vi "GeneratorBiasCurrents.vi"(10 "CurrentWaveForm":T1={"StartCurrent (mA)"=1.0, "MaximumCurrent (mA)"=3.0, "NumberOfCurrentPoints"=3, "NumberOfPointsInPulse"=20, "NumOfPointsAtPulseMAX"=4, "Exponent"=1, "CurrentStep (mA)"=1.0, "NumOfPointsAtPulseMIN"=8, "Next current step"=0.0} {"StartCurrent (mA)" min=0.001}) -> (0 "PulsedCurrentWaveForm":dbl[](array[numeric])=[0.0, 0.0, 0.0, 0.0, 0.0, 0.0, 0.0, 0.0, 0.0, 0.006819348298638839, 0.02709137914968268, 0.06026312439675552, 0.10542974530180321, 0.16135921418712945, 0.22652592093878654, 0.29915228767351526, 0.3772572564296004, 0.4587103272638338, 0.5412896727361661, 0.6227427435703996, 0.7008477123264847, 0.7734740790612133, 0.8386407858128705, 0.8945702546981968, 0.9397368756032445, 0.9729086208503173, 0.9931806517013612, 1.0, 1.0, 1.0, 1.0, 1.0, 1.0, 0.9931806517013612, 0.9729086208503173, 0.9397368756032445, 0.8945702546981968, 0.8386407858128706, 0.7734740790612135, 0.7008477123264847, 0.6227427435703996, 0.5412896727361662, 0.4587103272638339, 0.3772572564296004, 0.2991522876735153, 0.22652592093878665, 0.1613592141871295, 0.10542974530180316, 0.06026312439675552, 0.027091379149682737, 0.006819348298638839, 0.0, 0.0, 0.0, 0.0, 0.0, 0.0, 0.0, 0.0, 0.0, 0.0, 0.013638696597277677, 0.05418275829936536, 0.12052624879351104, 0.21085949060360643, 0.3227184283742589, 0.4530518418775731, 0.5983045753470305, 0.7545145128592008, 0.9174206545276676, 1.0825793454723323, 1.2454854871407992, 1.4016954246529694, 1.5469481581224267, 1.677281571625741, 1.7891405093963937, 1.879473751206489, 1.9458172417006345, 1.9863613034027223, 2.0, 2.0, 2.0, 2.0, 2.0, 2.0, 1.9863613034027223, 1.9458172417006345, 1.879473751206489, 1.7891405093963937, 1.6772815716257412, 1.546948158122427, 1.4016954246529694, 1.2454854871407992, 1.0825793454723325, 0.9174206545276677, 0.7545145128592008, 0.5983045753470306, 0.4530518418775733, 0.322718428374259, 0.21085949060360631, 0.12052624879351104, 0.054182758299365474, 0.013638696597277677, 0.0, 0.0, 0.0, 0.0, 0.0, 0.0, 0.0, 0.0, 0.0, 0.0, 0.020458044895916516, 0.08127413744904805, 0.18078937319026656, 0.31628923590540964, 0.48407764256138835, 0.6795777628163596, 0.8974568630205457, 1.1317717692888012, 1.3761309817915015, 1.6238690182084983, 1.8682282307111988, 2.1025431369794543, 2.32042223718364, 2.5159223574386114, 2.6837107640945908, 2.8192106268097334, 2.918725862550952, 2.9795419551040836, 3.0, 3.0, 3.0, 3.0, 3.0, 3.0, 2.9795419551040836, 2.918725862550952, 2.8192106268097334, 2.6837107640945903, 2.515922357438612, 2.3204222371836405, 2.1025431369794543, 1.8682282307111988, 1.6238690182084985, 1.3761309817915017, 1.1317717692888012, 0.8974568630205457, 0.67957776281636, 0.48407764256138863, 0.31628923590540925, 0.18078937319026656, 0.08127413744904821, 0.020458044895916405, 0.0])   [LabVIEW 2015]
uses:
  Waveform parameters.ctl
panel:
  out "Waveform parameters out":T1={"StartCurrent (mA)"=1.0, "MaximumCurrent (mA)"=3.0, "NumberOfCurrentPoints"=3, "NumberOfPointsInPulse"=20, "NumOfPointsAtPulseMAX"=4, "Exponent"=1, "CurrentStep (mA)"=1.0, "NumOfPointsAtPulseMIN"=8, "Next current step"=0.0} {"StartCurrent (mA)" min=0.001}
  out "XY Graph":cluster{i32[], dbl[]}(graph)={[0, 1, 2, 3, 4, 5, 6, 7, 8, 9, 10, 11, 12, 13, 14, 15, 16, 17, 18, 19, 20, 21, 22, 23, 24, 25, 26, 27, 28, 29, 30, 31, 32, 33, 34, 35, 36, 37, 38, 39, 40, 41, 42, 43, 44, 45, 46, 47, 48, 49, 50, 51, 52, 53, 54, 55, 56, 57, 58, 59, 60, 61, 62, 63, 64, 65, 66, 67, 68, 69, 70, 71, 72, 73, 74, 75, 76, 77, 78, 79, 80, 81, 82, 83, 84, 85, 86, 87, 88, 89, 90, 91, 92, 93, 94, 95, 96, 97, 98, 99, 100, 101, 102, 103, 104, 105, 106, 107, 108, 109, 110, 111, 112, 113, 114, 115, 116, 117, 118, 119, 120, 121, 122, 123, 124, 125, 126, 127, 128, 129, 130, 131, 132, 133, 134, 135, 136, 137, 138, 139, 140, 141, 142, 143, 144, 145, 146, 147, 148, 149, 150, 151, 152, 153, 154, 155], [0.0, 0.0, 0.0, 0.0, 0.0, 0.0, 0.0, 0.0, 0.0, 0.006819348298638839, 0.02709137914968268, 0.06026312439675552, 0.10542974530180321, 0.16135921418712945, 0.22652592093878654, 0.29915228767351526, 0.3772572564296004, 0.4587103272638338, 0.5412896727361661, 0.6227427435703996, 0.7008477123264847, 0.7734740790612133, 0.8386407858128705, 0.8945702546981968, 0.9397368756032445, 0.9729086208503173, 0.9931806517013612, 1.0, 1.0, 1.0, 1.0, 1.0, 1.0, 0.9931806517013612, 0.9729086208503173, 0.9397368756032445, 0.8945702546981968, 0.8386407858128706, 0.7734740790612135, 0.7008477123264847, 0.6227427435703996, 0.5412896727361662, 0.4587103272638339, 0.3772572564296004, 0.2991522876735153, 0.22652592093878665, 0.1613592141871295, 0.10542974530180316, 0.06026312439675552, 0.027091379149682737, 0.006819348298638839, 0.0, 0.0, 0.0, 0.0, 0.0, 0.0, 0.0, 0.0, 0.0, 0.0, 0.013638696597277677, 0.05418275829936536, 0.12052624879351104, 0.21085949060360643, 0.3227184283742589, 0.4530518418775731, 0.5983045753470305, 0.7545145128592008, 0.9174206545276676, 1.0825793454723323, 1.2454854871407992, 1.4016954246529694, 1.5469481581224267, 1.677281571625741, 1.7891405093963937, 1.879473751206489, 1.9458172417006345, 1.9863613034027223, 2.0, 2.0, 2.0, 2.0, 2.0, 2.0, 1.9863613034027223, 1.9458172417006345, 1.879473751206489, 1.7891405093963937, 1.6772815716257412, 1.546948158122427, 1.4016954246529694, 1.2454854871407992, 1.0825793454723325, 0.9174206545276677, 0.7545145128592008, 0.5983045753470306, 0.4530518418775733, 0.322718428374259, 0.21085949060360631, 0.12052624879351104, 0.054182758299365474, 0.013638696597277677, 0.0, 0.0, 0.0, 0.0, 0.0, 0.0, 0.0, 0.0, 0.0, 0.0, 0.020458044895916516, 0.08127413744904805, 0.18078937319026656, 0.31628923590540964, 0.48407764256138835, 0.6795777628163596, 0.8974568630205457, 1.1317717692888012, 1.3761309817915015, 1.6238690182084983, 1.8682282307111988, 2.1025431369794543, 2.32042223718364, 2.5159223574386114, 2.6837107640945908, 2.8192106268097334, 2.918725862550952, 2.9795419551040836, 3.0, 3.0, 3.0, 3.0, 3.0, 3.0, 2.9795419551040836, 2.918725862550952, 2.8192106268097334, 2.6837107640945903, 2.515922357438612, 2.3204222371836405, 2.1025431369794543, 1.8682282307111988, 1.6238690182084985, 1.3761309817915017, 1.1317717692888012, 0.8974568630205457, 0.67957776281636, 0.48407764256138863, 0.31628923590540925, 0.18078937319026656, 0.08127413744904821, 0.020458044895916405, 0.0]}
  # "NumOfPointsAtPulseMax*2^(Exponent)=NumOfPointsAtPulseMIN"
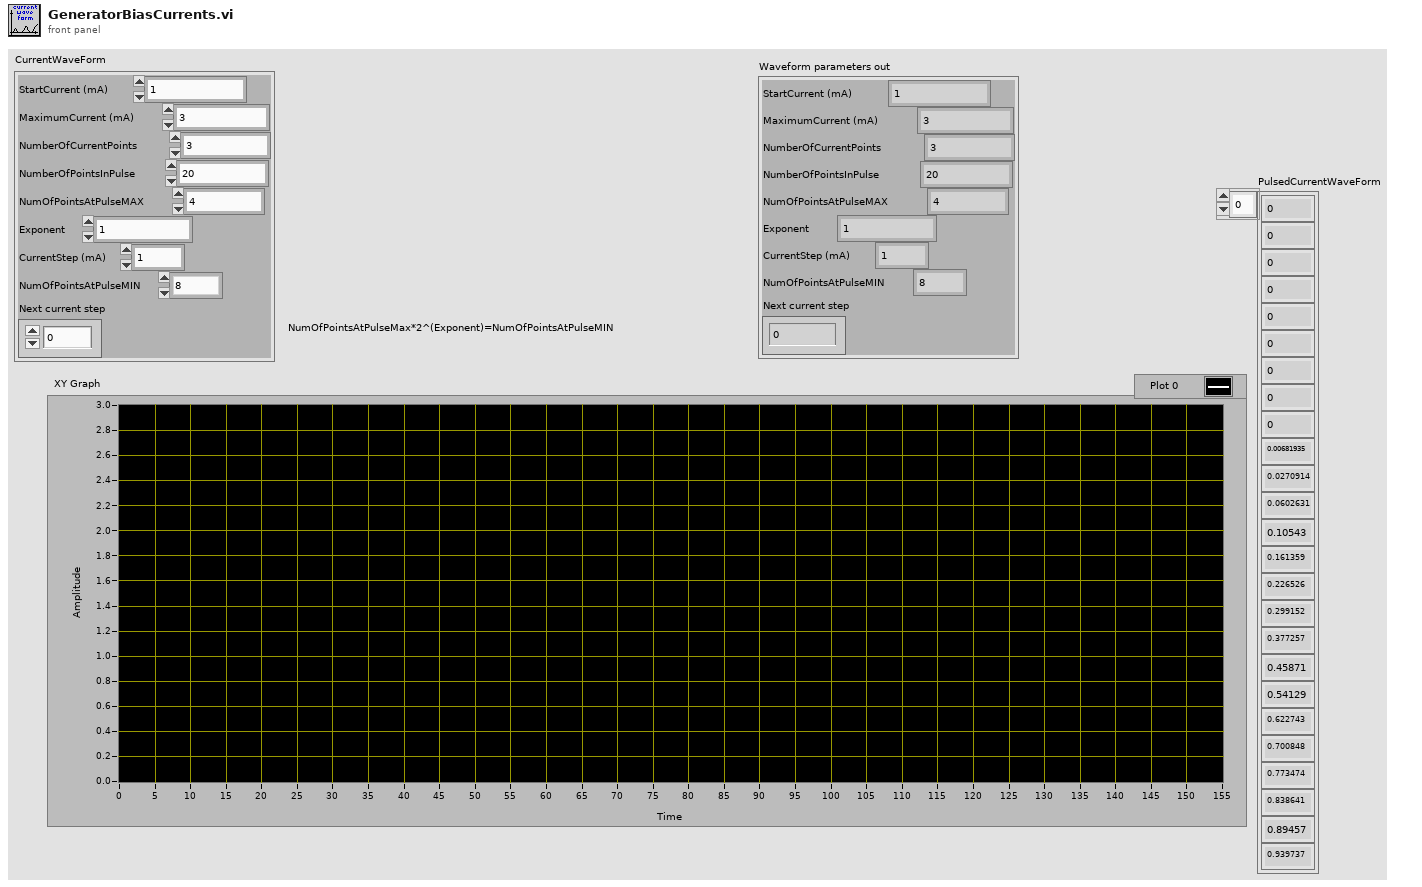
[diagram p1: front panel]
types:
  T1 = typedef "Waveform parameters.ctl" = cluster{"StartCurrent (mA)":dbl, "MaximumCurrent (mA)":dbl, "NumberOfCurrentPoints":i32, "NumberOfPointsInPulse":i32, "NumOfPointsAtPulseMAX":i32, "Exponent":i16, "CurrentStep (mA)":dbl, "NumOfPointsAtPulseMIN":i32, "Next current step":dbl}
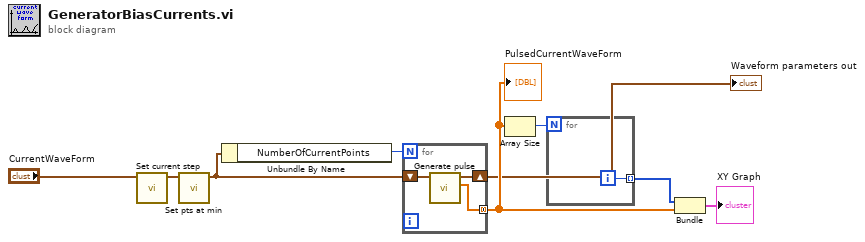
[diagram p0: block diagram]
diagram:
  n1 = call "Set current step.vi"("Waveform parameters"="CurrentWaveForm") -> ("Waveform parameters out"=w2:T1)  [unwired: 10 in]
  n2 = call "Set pts at min.vi"("Waveform parameters"=w2) -> ("Waveform parameters out"=w3:T1)  [unwired: 10 in]
  n3 = Unbundle By Name(w3) -> ("NumberOfCurrentPoints"=w4:i32)
  n4 = for {
    N: w4 -> [_]
    shift-right: [w11] -> w1
    shift-left: w3 -> [w12]
    tunnel: [w10] -> w5 mode=concatenating
    n5 = call "Generate pulse.vi"("Waveform parameters"=w12) -> ("Data out"=w10:dbl[], "Waveform parameters out"=w11:T1)  [unwired: 9 in]
  }
  "PulsedCurrentWaveForm" <- w5
  "Waveform parameters out" <- w1
  n6 = Array Size(array=w5) -> (size(s)=w8:i32)
  n7 = for {
    N: w8 -> [_]
    tunnel: [w13] -> w7 mode=indexing
    i -> [w13]
  }
  n8 = Bundle(w7, "Data out"=w5) -> (→"XY Graph":cluster{i32[], "Data out":dbl[]})  [unwired: 1 in]
